vi "Build Item Path.vi"(10 "Base Path":string, 11 "Item URL":string) -> (3 "Item Path":string)   [LabVIEW 2020, in "LV Project Items Parser.lvlib"]
doc: "Builds the absolute path for a given project items from its URL attribute."
uses:
  LV Project Items Parser.lvlib
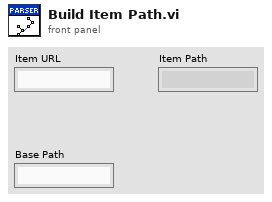
[diagram p1: front panel]
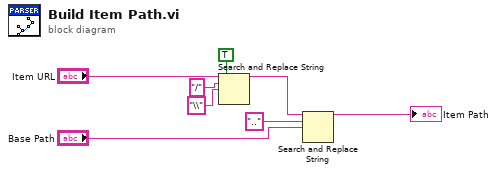
[diagram p0: block diagram]
diagram:
  n1 = Search and Replace String(replace all?=TRUE ("replace all? (F)"), input string="Item URL", search string="/", replace string="\\" ("replace string (\"\")")) -> (result string=w2:string)  [unwired: 4 in, 3 out]
  n2 = Search and Replace String(input string=w2, search string="..", replace string="Base Path") -> (result string=→"Item Path":string)  [unwired: 5 in, 3 out]
